vi "S2C_M2p5942_Proc_Commands.vi"(7 "VI_Ref":refnum<vi>, 8 "Error In":errorcluster, 10 "Settings":T1, 11 "Q-Ref":refnum<queue>) -> (0 "Error Out":errorcluster, 2 "Stop?":bool, 3 "Response":variant)   [LabVIEW 2024]
uses:
  S2C_M2p5942_Proc_Globals.vi
  _Shared/S2C_Shared_Proc_Globals.vi
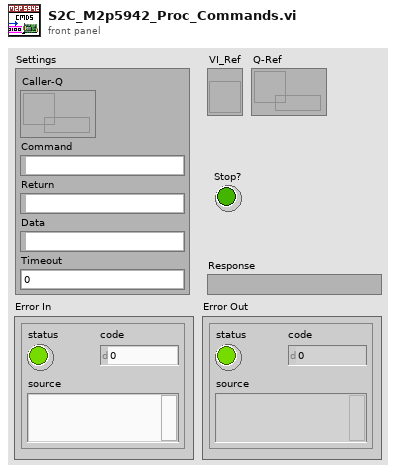
[diagram p1: front panel]
types:
  T1 = cluster{"Caller-Q":refnum<queue>, "Command":string, "Return":string, "Data":variant, "Timeout":dbl}
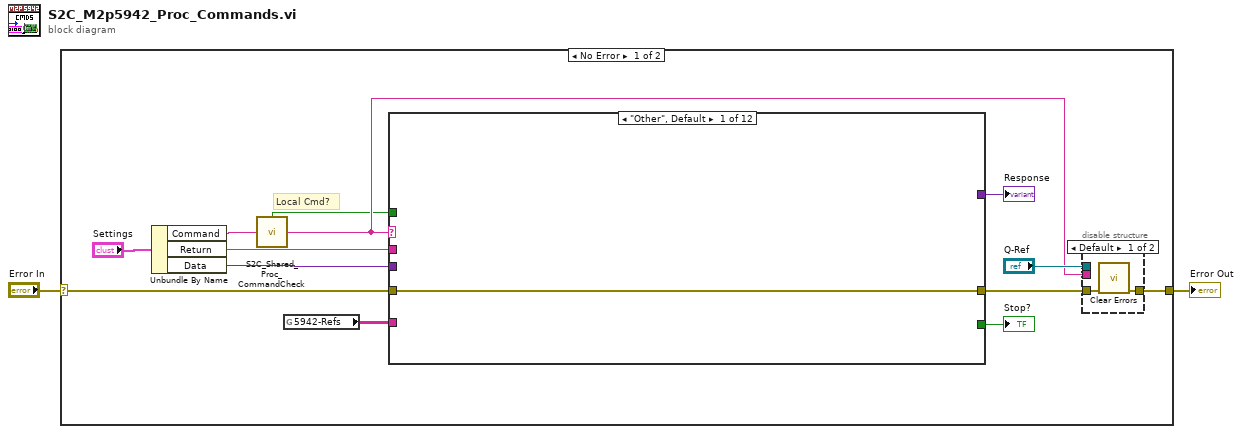
[diagram p0: block diagram]
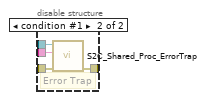
[diagram p2: hidden frame]
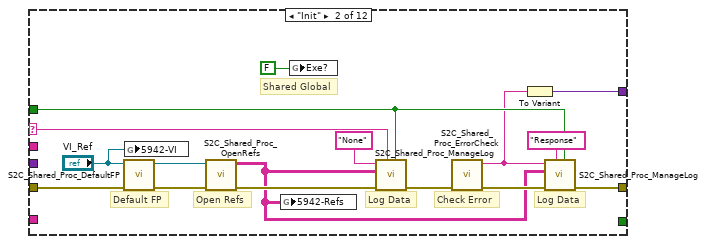
[diagram p3: hidden frame]
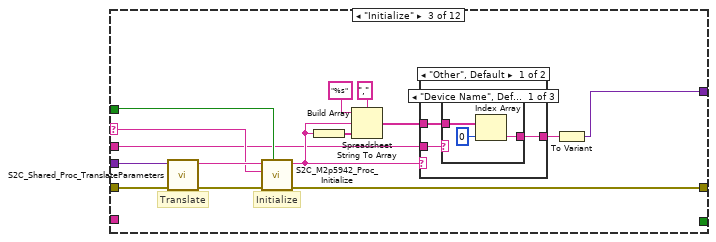
[diagram p4: hidden frame]
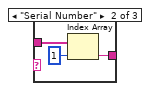
[diagram p5: hidden frame]
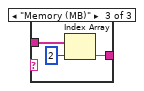
[diagram p6: hidden frame]
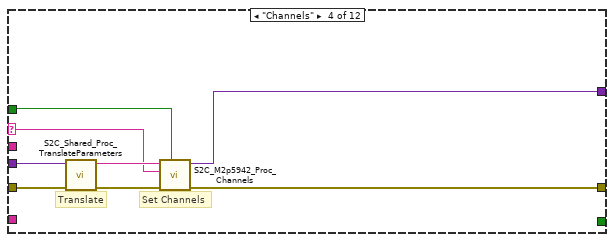
[diagram p8: hidden frame]
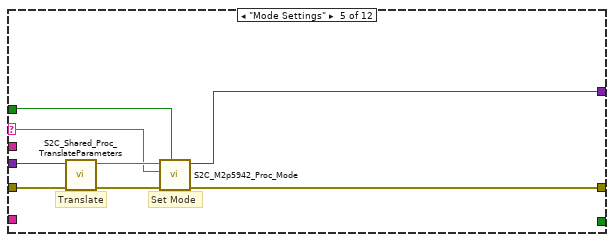
[diagram p9: hidden frame]
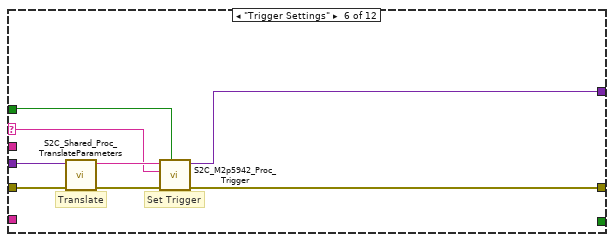
[diagram p10: hidden frame]
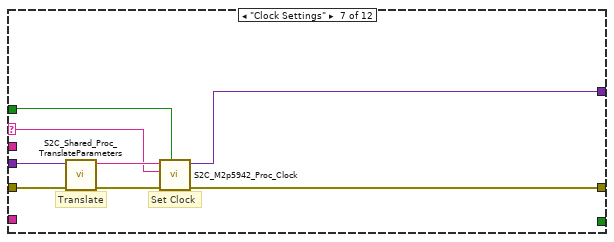
[diagram p11: hidden frame]
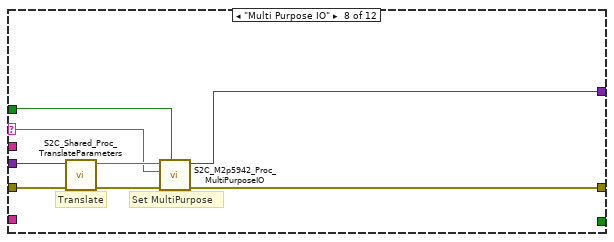
[diagram p12: hidden frame]
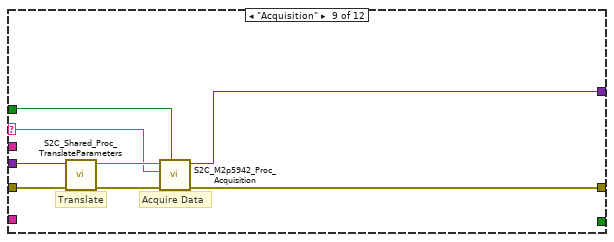
[diagram p13: hidden frame]
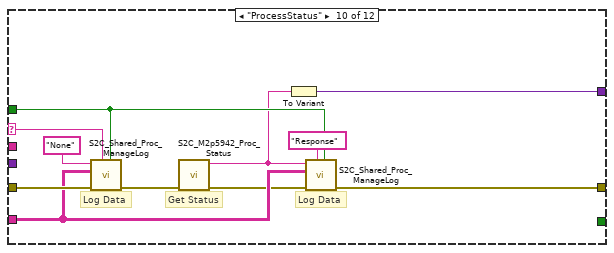
[diagram p14: hidden frame]
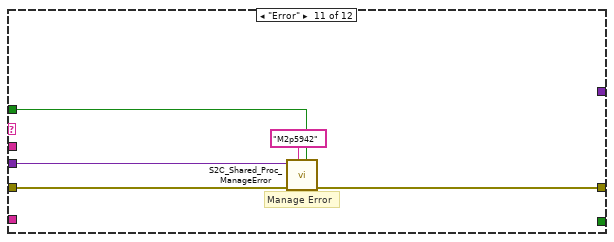
[diagram p15: hidden frame]
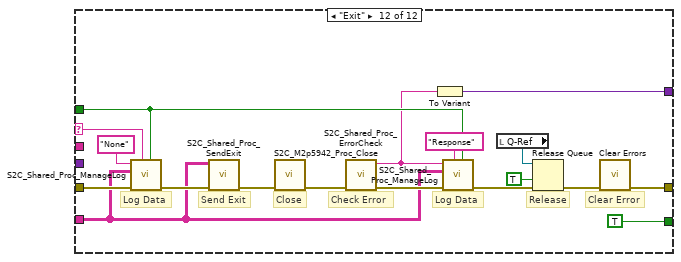
[diagram p16: hidden frame]
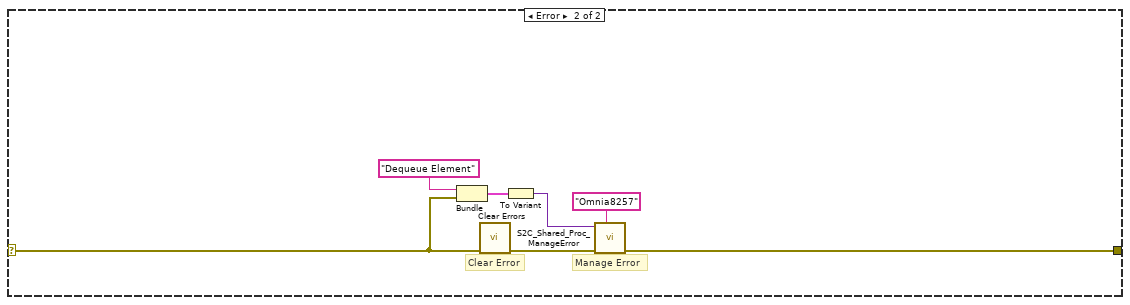
[diagram p17: hidden frame]
diagram:
  n1 = case shown="No Error" "Error In" {
    selector: "Error In" -> [w14 w150]
    tunnel: [w8 w149] -> w1
    frame No Error {
      # "Local Cmd?"
      n2 = Unbundle By Name("Settings") -> ("Command"=w6:string, "Return"=w10:string, "Data"=w15:variant)
      n3 = call "S2C_Shared_Proc_CommandCheck.vi"("Cmd In"=w6) -> ("Local?"=w4:bool, "Cmd Out"=w5:string)  [unwired: 13 in]
      n4 = global read "S2C_M2p5942_Proc_Globals.vi" "5942-Refs"() -> (w3:string[][])
      n5 = case shown="\"Other\", Default" w5 {
        selector: w5 -> [_ w35 w48 w69 w77 w85 w93 w101 w109 w124 _ w145]
        tunnel: w14 -> [w22 w27 w53 w74 w82 w90 w98 w106 w114 w123 w130 w146]
        tunnel: w15 -> [_ _ w52 w73 w81 w89 w97 w105 w113 _ w128 _]
        tunnel: [w22 w38 w47 w68 w76 w84 w92 w100 w108 w119 w129 w133] -> w9
        tunnel: [_ w32 w39 w67 w75 w83 w91 w99 w107 w120 _ w140] -> w12
        tunnel: [_ _ _ _ _ _ _ _ _ _ _ TRUE] -> w11
        tunnel: w10 -> [_ _ w42 _ _ _ _ _ _ _ _ _]
        tunnel: w4 -> [_ w36 w50 w71 w79 w87 w95 w103 w111 w122 w126 w144]
        tunnel: w3 -> [_ _ _ _ _ _ _ _ _ w118 _ w137]
        frame "Other", Default {
        }
        frame "Init" {
          # "Default FP"
          # "Shared Global"
          # "Check Error"
          # "Log Data"
          # "Open Refs"
          # "Log Data"
          n6 = call "S2C_Shared_Proc_DefaultFP.vi"("Error In"=w27, "VI_Ref In"="VI_Ref") -> ("Error Out"=w25:errorcluster, "VI_Ref Out"=w26:refnum<vi>)  [unwired: 8 in]
          n7 = global write "S2C_M2p5942_Proc_Globals.vi" "5942-VI"("VI_Ref") -> ()
          n8 = call "S2C_Shared_Proc_OpenRefs.vi"("Error In"=w25, "VI_Ref"=w26) -> ("Error Out"=w28:errorcluster, "Refs"=w23:string[][])  [unwired: 8 in]
          n9 = global write "S2C_M2p5942_Proc_Globals.vi" "5942-Refs"(w23) -> ()
          n10 = global write "S2C_Shared_Proc_Globals.vi" "Exe?"(FALSE ("Exe?")) -> ()
          n11 = call "S2C_Shared_Proc_ManageLog.vi"("Local?"=w36, "Command"=w35, "Error In"=w28, "Refs"=w23, "Data In"="None") -> ("Error Out"=w30:errorcluster)  [unwired: 5 in, 1 out]
          n12 = call "S2C_Shared_Proc_ErrorCheck.vi"("Error In"=w30) -> ("Error Out"=w33:errorcluster, "Status"=w31:string)  [unwired: 9 in]
          n13 = To Variant(anything=w31) -> (Variant=w32:variant)
          n14 = call "S2C_Shared_Proc_ManageLog.vi"("Local?"=w36, "Command"="Response", "Error In"=w33, "Refs"=w23, "Data In"=w31) -> ("Error Out"=w38:errorcluster)  [unwired: 5 in, 1 out]
        }
        frame "Initialize" {
          # "Initialize"
          # "Translate"
          n15 = call "S2C_Shared_Proc_TranslateParameters.vi"("Error In"=w53, "Data"=w52) -> ("Error Out"=w51:errorcluster, "JSON Cluster"=w49:string)  [unwired: 8 in]
          n16 = call "S2C_M2p5942_Proc_Initialize.vi"("Local?"=w50, "Error In"=w51, "Command"=w48, "JSON String"=w49) -> ("Error Out"=w47:errorcluster, "Response"=w43:string)  [unwired: 6 in]
          n17 = Build Array(w43) -> (w44:string[])
          n18 = Spreadsheet String To Array(delimiter (Tab)=",", format string="%s", spreadsheet string=w43, array type (2D Dbl)=w44) -> (array=w41:string[])
          n19 = case shown="\"Other\", Default" w43 {
            selector: w43 -> [_ w66]
            tunnel: w42 -> [w56 _]
            tunnel: w41 -> [w55 _]
            tunnel: [w54 w66] -> w40
            frame "Other", Default {
              n20 = case shown="\"Device Name\", Default" w56 {
                tunnel: w55 -> [w59 w62 w65]
                tunnel: [w57 w60 w63] -> w54
                frame "Device Name", Default {
                  n21 = Index Array(array=w59, index=0) -> (element=w57:string)
                }
                frame "Serial Number" {
                  n22 = Index Array(array=w62, index=1) -> (element=w60:string)
                }
                frame "Memory (MB)" {
                  n23 = Index Array(array=w65, index=2) -> (element=w63:string)
                }
              }
            }
            frame "Error" {
            }
          }
          n24 = To Variant(anything=w40) -> (Variant=w39:variant)
        }
        frame "Channels" {
          # "Set Channels"
          # "Translate"
          n25 = call "S2C_Shared_Proc_TranslateParameters.vi"("Error In"=w74, "Data"=w73) -> ("Error Out"=w72:errorcluster, "JSON Cluster"=w70:string)  [unwired: 8 in]
          n26 = call "S2C_M2p5942_Proc_Channels.vi"("Local?"=w71, "Error In"=w72, "Command"=w69, "JSON String"=w70) -> ("Error Out"=w68:errorcluster, "Response"=w67:variant)  [unwired: 6 in]
        }
        frame "Mode Settings" {
          # "Set Mode"
          # "Translate"
          n27 = call "S2C_Shared_Proc_TranslateParameters.vi"("Error In"=w82, "Data"=w81) -> ("Error Out"=w80:errorcluster, "JSON Cluster"=w78:string)  [unwired: 8 in]
          n28 = call "S2C_M2p5942_Proc_Mode.vi"("Local?"=w79, "Error In"=w80, "Command"=w77, "JSON String"=w78) -> ("Error Out"=w76:errorcluster, "Response"=w75:variant)  [unwired: 6 in]
        }
        frame "Trigger Settings" {
          # "Set Trigger"
          # "Translate"
          n29 = call "S2C_Shared_Proc_TranslateParameters.vi"("Error In"=w90, "Data"=w89) -> ("Error Out"=w88:errorcluster, "JSON Cluster"=w86:string)  [unwired: 8 in]
          n30 = call "S2C_M2p5942_Proc_Trigger.vi"("Local?"=w87, "Error In"=w88, "Command"=w85, "JSON String"=w86) -> ("Error Out"=w84:errorcluster, "Response"=w83:variant)  [unwired: 6 in]
        }
        frame "Clock Settings" {
          # "Set Clock"
          # "Translate"
          n31 = call "S2C_Shared_Proc_TranslateParameters.vi"("Error In"=w98, "Data"=w97) -> ("Error Out"=w96:errorcluster, "JSON Cluster"=w94:string)  [unwired: 8 in]
          n32 = call "S2C_M2p5942_Proc_Clock.vi"("Local?"=w95, "Error In"=w96, "Command"=w93, "JSON String"=w94) -> ("Error Out"=w92:errorcluster, "Response"=w91:variant)  [unwired: 6 in]
        }
        frame "Multi Purpose IO" {
          # "Set MultiPurpose"
          # "Translate"
          n33 = call "S2C_Shared_Proc_TranslateParameters.vi"("Error In"=w106, "Data"=w105) -> ("Error Out"=w104:errorcluster, "JSON Cluster"=w102:string)  [unwired: 8 in]
          n34 = call "S2C_M2p5942_Proc_MultiPurposeIO.vi"("Local?"=w103, "Error In"=w104, "Command"=w101, "JSON String"=w102) -> ("Error Out"=w100:errorcluster, "Response"=w99:variant)  [unwired: 6 in]
        }
        frame "Acquisition" {
          # "Acquire Data"
          # "Translate"
          n35 = call "S2C_Shared_Proc_TranslateParameters.vi"("Error In"=w114, "Data"=w113) -> ("Error Out"=w112:errorcluster, "JSON Cluster"=w110:string)  [unwired: 8 in]
          n36 = call "S2C_M2p5942_Proc_Acquisition.vi"("Local?"=w111, "Error In"=w112, "Command"=w109, "JSON String"=w110) -> ("Error Out"=w108:errorcluster, "Response"=w107:variant)  [unwired: 6 in]
        }
        frame "ProcessStatus" {
          # "Get Status"
          # "Log Data"
          # "Log Data"
          n37 = call "S2C_Shared_Proc_ManageLog.vi"("Local?"=w122, "Command"=w124, "Error In"=w123, "Refs"=w118, "Data In"="None") -> ("Error Out"=w117:errorcluster)  [unwired: 5 in, 1 out]
          n38 = call "S2C_M2p5942_Proc_Status.vi"("Error In"=w117) -> ("Error Out"=w116:errorcluster, "Response"=w115:string)  [unwired: 9 in]
          n39 = To Variant(anything=w115) -> (Variant=w120:variant)
          n40 = call "S2C_Shared_Proc_ManageLog.vi"("Local?"=w122, "Command"="Response", "Error In"=w116, "Refs"=w118, "Data In"=w115) -> ("Error Out"=w119:errorcluster)  [unwired: 5 in, 1 out]
        }
        frame "Error" {
          # "Manage Error"
          n41 = call "S2C_Shared_Proc_ManageError.vi"("Local?"=w126, "Process"="M2p5942", "Error In"=w130, "Data"=w128) -> ("Error Out"=w129:errorcluster)  [unwired: 7 in]
        }
        frame "Exit" {
          # "Close"
          # "Clear Error"
          # "Release"
          # "Check Error"
          # "Send Exit"
          # "Log Data"
          # "Log Data"
          n42 = call "S2C_Shared_Proc_ManageLog.vi"("Local?"=w144, "Command"=w145, "Error In"=w146, "Refs"=w137, "Data In"="None") -> ("Error Out"=w138:errorcluster)  [unwired: 5 in, 1 out]
          n43 = call "S2C_Shared_Proc_SendExit.vi"("Error In"=w138, "Refs"=w137) -> ("Error Out"=w132:errorcluster)  [unwired: 9 in]
          n44 = call "S2C_M2p5942_Proc_Close.vi"("Error In"=w132) -> ("Error Out"=w131:errorcluster)  [unwired: 10 in]
          n45 = call "S2C_Shared_Proc_ErrorCheck.vi"("Error In"=w131) -> ("Error Out"=w142:errorcluster, "Status"=w139:string)  [unwired: 9 in]
          n46 = To Variant(anything=w139) -> (Variant=w140:variant)
          n47 = call "S2C_Shared_Proc_ManageLog.vi"("Local?"=w144, "Command"="Response", "Error In"=w142, "Refs"=w137, "Data In"=w139) -> ("Error Out"=w141:errorcluster)  [unwired: 5 in, 1 out]
          n48 = local read "Q-Ref"() -> (w135:refnum<queue>)
          n49 = Release Queue(queue=w135, force destroy? (F)=TRUE, error in (no error)=w141) -> (error out=w136:errorcluster)  [unwired: 2 out]
          n50 = call <vilib>:"Clear Errors.vi"("error in (no error)"=w136) -> ("error out"=w133:errorcluster)  [unwired: 5 in, 1 out]
        }
      }
      "Response" <- w12
      "Stop?" <- w11
      n51 = disable-structure shown="Default" {
        disable-tunnel: w9 -> [w17 w21]
        disable-tunnel: [w16 w20] -> w8
        disable-tunnel: w5 -> [_ w19]
        disable-tunnel: "Q-Ref" -> [_ w18]
        frame condition #0 (active) {
          n52 = call <vilib>:"Clear Errors.vi"("error in (no error)"=w17) -> ("error out"=w16:errorcluster)  [unwired: 5 in, 1 out]
        }
        frame condition #1 {
          # "Error Trap"
          n53 = call "S2C_Shared_Proc_ErrorTrap.vi"("Error In"=w21, "Command"=w19, "Q-Ref"=w18) -> ("Error Out"=w20:errorcluster)  [unwired: 8 in]
        }
      }
    }
    frame Error {
      # "Clear Error"
      # "Manage Error"
      n54 = Bundle("Dequeue Element", "error IO"=w150) -> (w154:cluster{string, "error IO":errorcluster})  [unwired: 1 in]
      n55 = call <vilib>:"Clear Errors.vi"("error in (no error)"=w150) -> ("error out"=w151:errorcluster)  [unwired: 5 in, 1 out]
      n56 = To Variant(anything=w154) -> (Variant=w152:variant)
      n57 = call "S2C_Shared_Proc_ManageError.vi"("Process"="Omnia8257", "Error In"=w151, "Data"=w152) -> ("Error Out"=w149:errorcluster)  [unwired: 8 in]
    }
  }
  "Error Out" <- w1
